vi "Array Control Enable.vi"(8 "error in":errorcluster, 10 "Array Control in":refnum<vi>[](array[refnum])) -> (0 "error out":errorcluster)   [LabVIEW 2025, in "_Shared.lvlib"]
uses:
  _Shared.lvlib
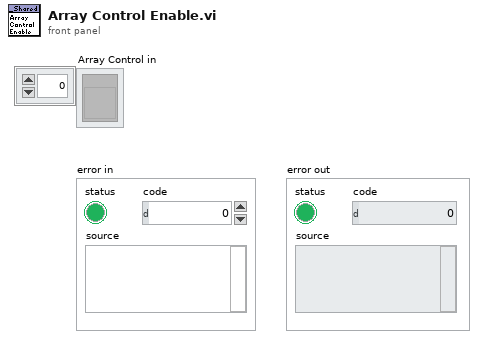
[diagram p1: front panel]
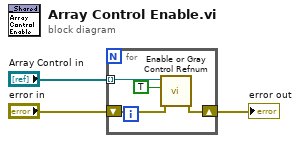
[diagram p0: block diagram]
diagram:
  n1 = for {
    tunnel: "Array Control in" -> [w4] mode=indexing
    shift-right: [w5] -> w2
    shift-left: "error in" -> [w6]
    n2 = call <vilib>:"Enable or Gray Control Refnum.vi"("error in (no error)"=w6, "enable?"=TRUE, "Control in"=w4) -> ("error out"=w5:errorcluster)  [unwired: 7 in, 1 out]
  }
  "error out" <- w2
